vi "Timer.vi"(3 "error in (no error)":errorcluster, 4 "Timer Value":dbl, 5 "timer_ops":T1) -> (0 "error out":errorcluster, 1 "Timer Done?":bool, 2 "Time Elasped":dbl)   [LabVIEW 2013]
uses:
  timer.ctl
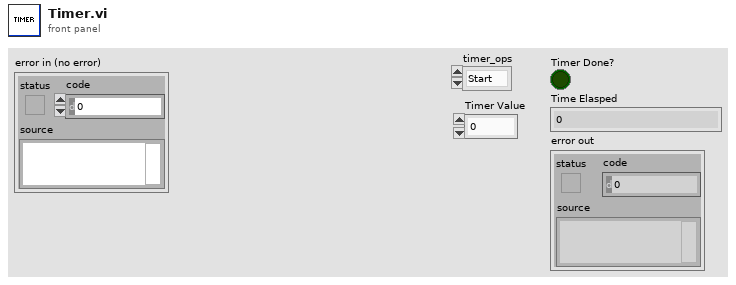
[diagram p1: front panel]
types:
  T1 = typedef "timer.ctl" = enum16{"Start", "Read"}
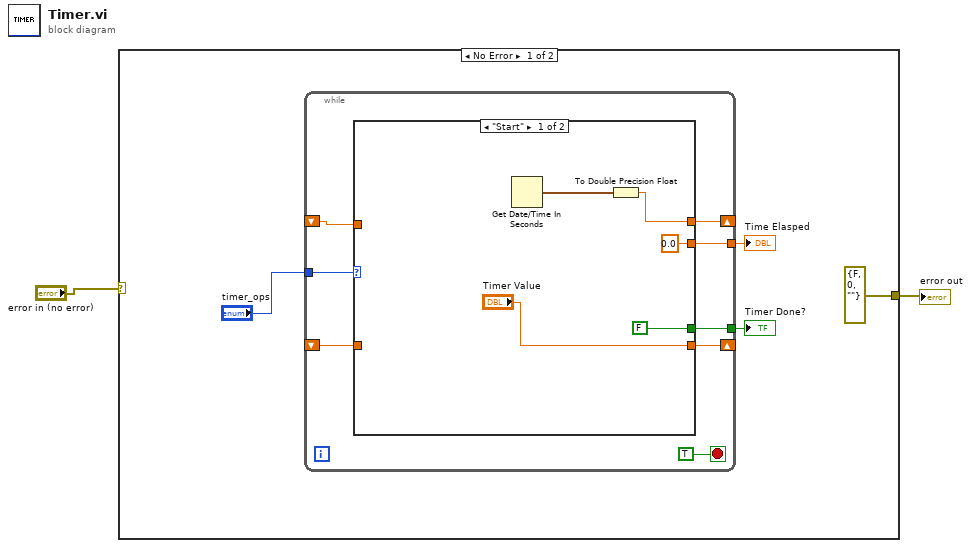
[diagram p0: block diagram]
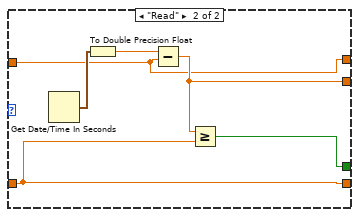
[diagram p2: hidden frame]
diagram:
  n1 = case shown="No Error" "error in (no error)" {
    selector: "error in (no error)" -> [_ w26]
    tunnel: [errorcluster {"status"=FALSE, "code"=0, "source"=""} ("error in (no error)") w26] -> w1
    frame No Error {
      n2 = while {
        tunnel: "timer_ops" -> [w14]
        tunnel: [w11] -> w5
        tunnel: [w10] -> w4
        shift-right: [w9] -> _
        shift-left: _ -> [w12]
        shift-right: [w8] -> _
        shift-left: _ -> [w7]
        stop <- TRUE stop-if-true
        n3 = case shown="\"Start\"" w14 {
          tunnel: w12 -> [_ w22]
          tunnel: [FALSE w24] -> w11
          tunnel: [0.0 w25] -> w10
          tunnel: ["Timer Value" w22] -> w9
          tunnel: [w16 w20] -> w8
          tunnel: w7 -> [_ w20]
          frame "Start" {
            n4 = Get Date/Time In Seconds() -> (seconds since 1Jan1904=w18:timestamp)
            n5 = To Double Precision Float(number=w18) -> (double precision float=w16:dbl)
          }
          frame "Read" {
            n6 = Get Date/Time In Seconds() -> (seconds since 1Jan1904=w23:timestamp)
            n7 = To Double Precision Float(number=w23) -> (double precision float=w21:dbl)
            n8 = Subtract(x=w21, y=w20) -> (x-y=w25:dbl)
            n9 = Greater Or Equal?(x=w25, y=w22) -> (x >= y?=w24:bool)
          }
        }
      }
      "Timer Done?" <- w5
      "Time Elasped" <- w4
    }
    frame Error {
    }
  }
  "error out" <- w1
